vi "On Line Calibration test.vi"(8 "error in (no error)":errorcluster, 10 "Session In":T1="cam1", 11 "Dove salvo l'immagine Calib Info":path=path "C:/Users/Dell/Documents/UNIVERSITA'/SistemiDiVisione/LabView/On Line calibration/calib-info.png") -> (0 "error out":errorcluster, 3 "Calibration Axis Info":T4={"Origin Pixel"={"X"=44.15415, "Y"=79.22556}, "Angle Relative to Horizontal (deg)"=0.0, "X Axis Pixel"={"X"=0.0, "Y"=0.0}, "Axis Reference"=1} {"X Axis Pixel"."Y" format="%.2f"; "X Axis Pixel"."X" format="%.2f"; "Axis Reference" items=["Direct", "Indirect"]; "Angle Relative to Horizontal (deg)" format="%.2f"; "Origin Pixel"."Y" format="%.2f"; "Origin Pixel"."X" format="%.2f"})   [LabVIEW 2020]
uses:
  <vilib>/vision/Calibration.llb/Error Statistics.ctl
  <vilib>/userdefined/High Color/IMAQdx.ctl
  <vilib>/vision/driver/NI_Vision_Acquisition_Software.lvlib
  <vilib>/vision/NI_Vision_Development_Module.lvlib
panel:
  in  "pulire memorie?":bool
  out "Error Map":sgl[][](array[numeric]) format="%.2f"
  out "Error Statistics":T2
  in  "Grid Descriptor 2":cluster{"X Step":sgl, "Y Step":sgl, "Unit":T3}={"X Step"=10.0, "Y Step"=10.0, "Unit"=enum."Millimeter"}
  out "Preprocessed image":T5(plugin-control)
  out "Input Calibration Grid":T5(plugin-control)
  in  "Stop Acquisizione":bool
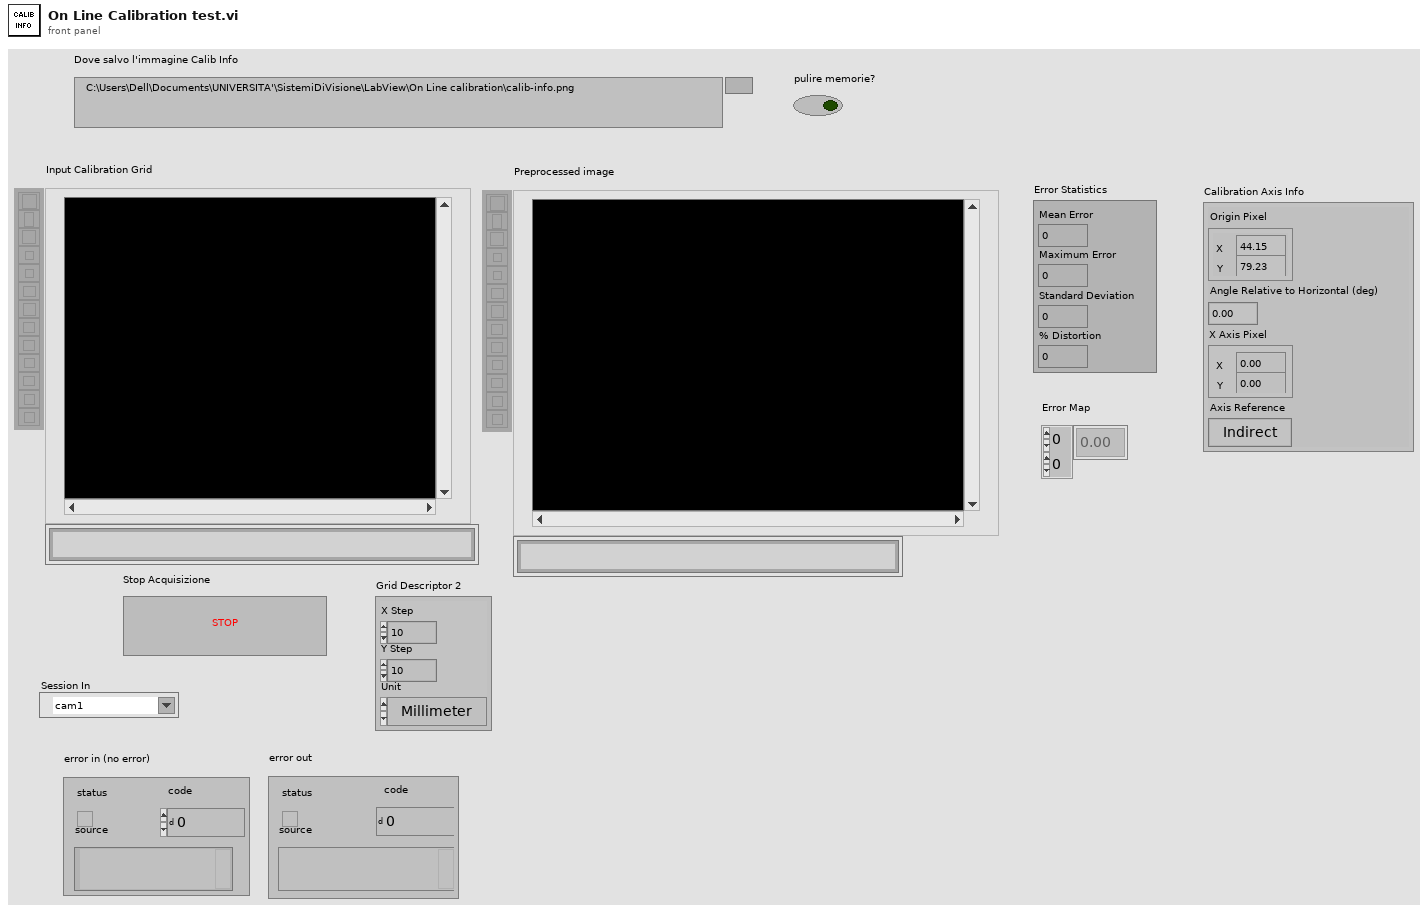
[diagram p1: front panel]
types:
  T1 = typedef "IMAQdx.ctl" = refnum<k21>
  T2 = typedef "Error Statistics.ctl" = cluster{"Mean Error":dbl, "Maximum Error":dbl, "Standard Deviation":dbl, "% Distortion":dbl}
  T3 = typedef "Image Unit" = enum32{"Undefined", "Angström", "Micrometer", "Millimeter", "Centimeter", "Meter", "Kilometer", "Microinch", "Inch", "Feet", "Nautical miles", "Standard miles", "Steps"}
  T4 = cluster{"Origin Pixel":cluster{"X":sgl, "Y":sgl}, "Angle Relative to Horizontal (deg)":sgl, "X Axis Pixel":cluster{"X":sgl, "Y":sgl}, "Axis Reference":u32}
  T5 = typedef "IMAQ Image.ctl" = refnum<image>
  T6 = typedef "Image Type" = u32
  T7 = typedef "Calibration Reference Points.ctl" = cluster{"Pixel Coordinates":cluster{"X":dbl, "Y":dbl}[], "Real World Coordinates":cluster{"X":dbl, "Y":dbl}[], "Unit":T3, "Image Size":cluster{"X":u32, "Y":u32}}
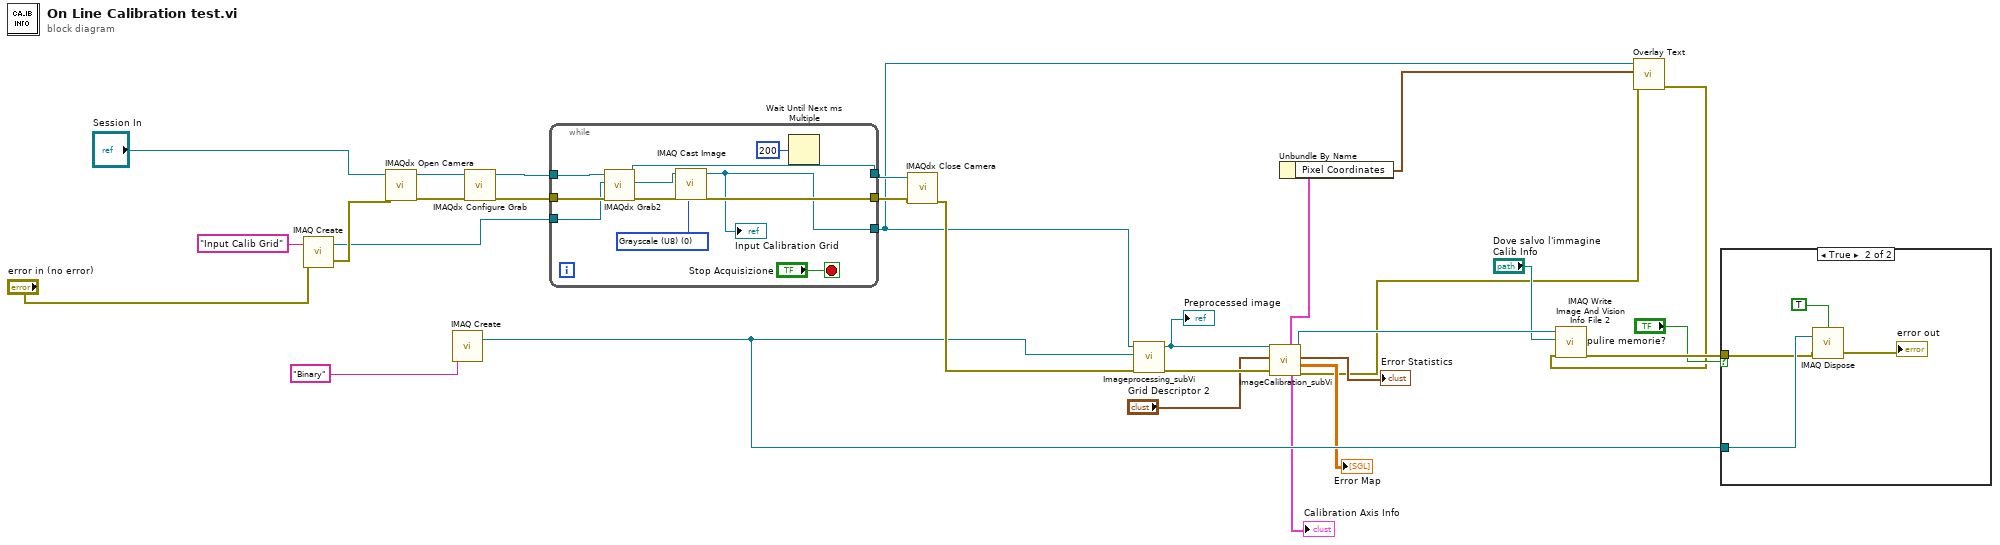
[diagram p0: block diagram]
diagram:
  n1 = call "IMAQ Create"("Image Name"="Input Calib Grid", "error in (no error)"="error in (no error)") -> ("New Image"=w19:T5, "error out"=w22:errorcluster)  [unwired: 3 in]
  n2 = call <vilib>:"IMAQdx Open Camera.vi"("error in"=w22, "Session In"="Session In") -> ("error out"=w24:errorcluster, "Session Out"=w26:T1)  [unwired: 8 in]
  n3 = call "IMAQ Create"("Image Name"="Binary") -> ("New Image"=w17:T5)  [unwired: 4 in, 1 out]
  n4 = call <vilib>:"IMAQdx Configure Grab.vi"("error in"=w24, "Session In"=w26) -> ("error out"=w23:errorcluster, "Session Out"=w27:T1)  [unwired: 8 in]
  n5 = while {
    tunnel: w19 -> [w31]
    tunnel: w27 -> [w37]
    tunnel: w23 -> [w36]
    tunnel: [w35] -> w21
    tunnel: [w34] -> w20
    tunnel: [w32] -> w2
    stop <- "Stop Acquisizione" stop-if-true
    w30 = T6 0 items=["Grayscale (U8)", "Grayscale (I16)", "Grayscale (SGL)", "Complex (CSG)", "RGB (U32)", "HSL (U32)", "RGB (U64)", "Grayscale (U16)"] ("Image Type")
    n6 = call <vilib>:"IMAQdx Grab2.vi"("error in"=w36, "Image In"=w31, "Session In"=w37) -> ("error out"=w34:errorcluster, "Image Out"=w33:T5, "Session Out"=w35:T1)  [unwired: 5 in, 1 out]
    n7 = call "IMAQ Cast Image"("Image Type"=w30, "Image Src"=w33) -> ("Image Dst Out"=w32:T5)  [unwired: 8 in, 1 out]
    "Input Calibration Grid" <- w32
    n8 = Wait Until Next ms Multiple(millisecond multiple=u32 200) -> ()  [unwired: 1 out]
  }
  n9 = call <vilib>:"IMAQdx Close Camera.vi"("error in"=w20, "Session In"=w21) -> ("error out"=w18:errorcluster)  [unwired: 9 in]
  n10 = call "Imageprocessing_subVi.vi"("error in (no error)"=w18, "Binary Img"=w17, "Image In"=w2) -> ("error out"=w16:errorcluster, "Image Dst Out"=w14:T5)  [unwired: 7 in]
  "Preprocessed image" <- w14
  n11 = call "ImageCalibration_subVi.vi"("error in (no error)"=w16, "Grid Descriptor"="Grid Descriptor 2", "Preprocedded Img In"=w14) -> ("error out"=w4:errorcluster, "Error Map"=→"Error Map":sgl[][], "Error Statistics"=→"Error Statistics":T2, "Calibration Template Image (duplicate)"=w8:T5, "Calibration Axis Info"=→"Calibration Axis Info":T4, "Reference Points"=w10:T7)  [unwired: 3 in]
  n12 = Unbundle By Name(w10) -> ("Pixel Coordinates"=w1:cluster{"X":dbl, "Y":dbl}[])
  n13 = call "Overlay Text.vi"("error in (no error)"=w4, "Pixel Coordinates"=w1, "Refnum in"=w2) -> ("error out"=w3:errorcluster)  [unwired: 8 in]
  n14 = call "IMAQ Write Image And Vision Info File 2"("error in (no error)"=w3, "File Path"="Dove salvo l'immagine Calib Info", "Image"=w8) -> ("error out"=w7:errorcluster)  [unwired: 7 in, 1 out]
  n15 = case shown="True" "pulire memorie?" {
    tunnel: w17 -> [_ w43]
    tunnel: w7 -> [_ w41]
    frame False {
    }
    frame True {
      n16 = call "IMAQ Dispose"("All Images? (No)"=TRUE, "Image"=w43, "error in (no error)"=w41) -> ("error out"=→"error out":errorcluster)  [unwired: 3 in]
    }
  }
